vi "Pet Keepalive.vi"(7 "Server Alias":string, 8 "error in (no error)":errorcluster) -> (0 "error out":errorcluster)   [LabVIEW 2013, in "TS.lvlib"]
doc: "This VI \"pets\" the internal keep-alive in the Server.vi. So if the LabVIEW side goes down, the Server.vi will go down."
uses:
  TS.lvlib
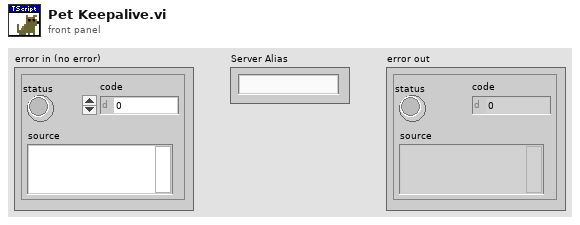
[diagram p1: front panel]
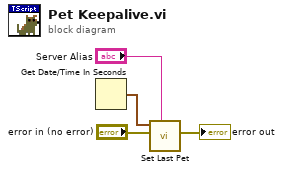
[diagram p0: block diagram]
diagram:
  n1 = Get Date/Time In Seconds() -> (seconds since 1Jan1904=w2:timestamp)
  n2 = call "Set Last Pet.vi"("Server Alias"="Server Alias", "Error In"="error in (no error)", "Last Pet"=w2) -> ("Error Out"=→"error out":errorcluster)  [unwired: 8 in]
